vi "GUI_PhasicsHPD.vi"() -> ()   [LabVIEW 2013]
uses:
  shared programs/GUI_Template/GUI_master/tcp_new_data_event.ctl
  shared programs/GUI_Template/GUI_master/tcp new data cluster.ctl
  <vilib>/vision/NI_Vision_Development_Module.lvlib
panel:
  out "Overexposed!":bool
  in  "Tab Control":enum32{"Raw", "Intensity", "Phase"}(tab)
  out "image::1":T1(plugin-control) caption="Raw"
  out "intensityimage::1":T1(plugin-control) caption="Intensity"
  out "phaseimage::1":T1(plugin-control) caption="Phase"
  in  "gain::1":dbl=0.001 caption="gain" min=0.451 max=21.5 format="%_4p"
  in  "exposure::1":dbl=0.001 caption="Exposure" min=0.001 max=1.0 format="%_4p"
  in  "insert tag":bool=TRUE
  in  "stop":bool
  in  "trigger::1":bool caption="Trigger"
  in  "GUIdevice 1":string="U_Phasics"
  out "tcp data event":T2
  out "error IO 2":errorcluster
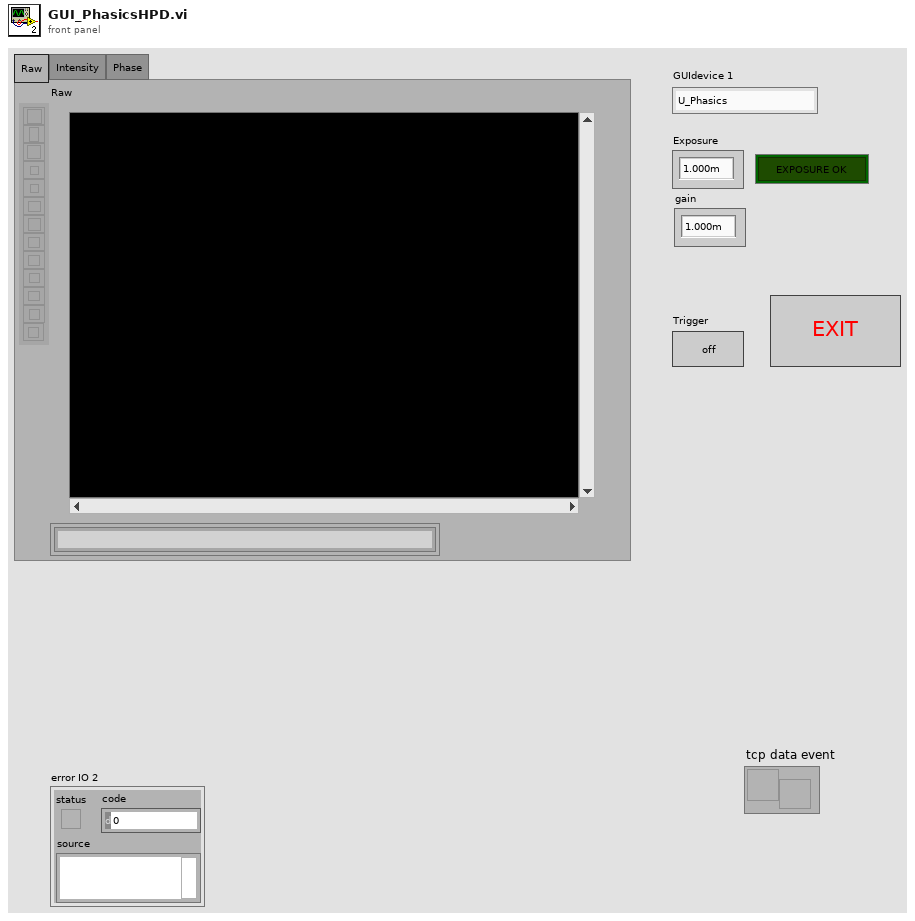
[diagram p1: front panel]
types:
  T1 = typedef "IMAQ Image.ctl" = refnum<image>
  T2 = typedef "tcp_new_data_event.ctl" = refnum<user-event>
  T3 = typedef "Image Type" = u32
  T4 = typedef "tcp new data cluster.ctl" = cluster{"EventEnum":enum16{"new data", "connection status update"}, "Device name":string}
  T5 = cluster{"Starting Value":sgl, "Incremental Value":sgl, "Histogram":u32[]}
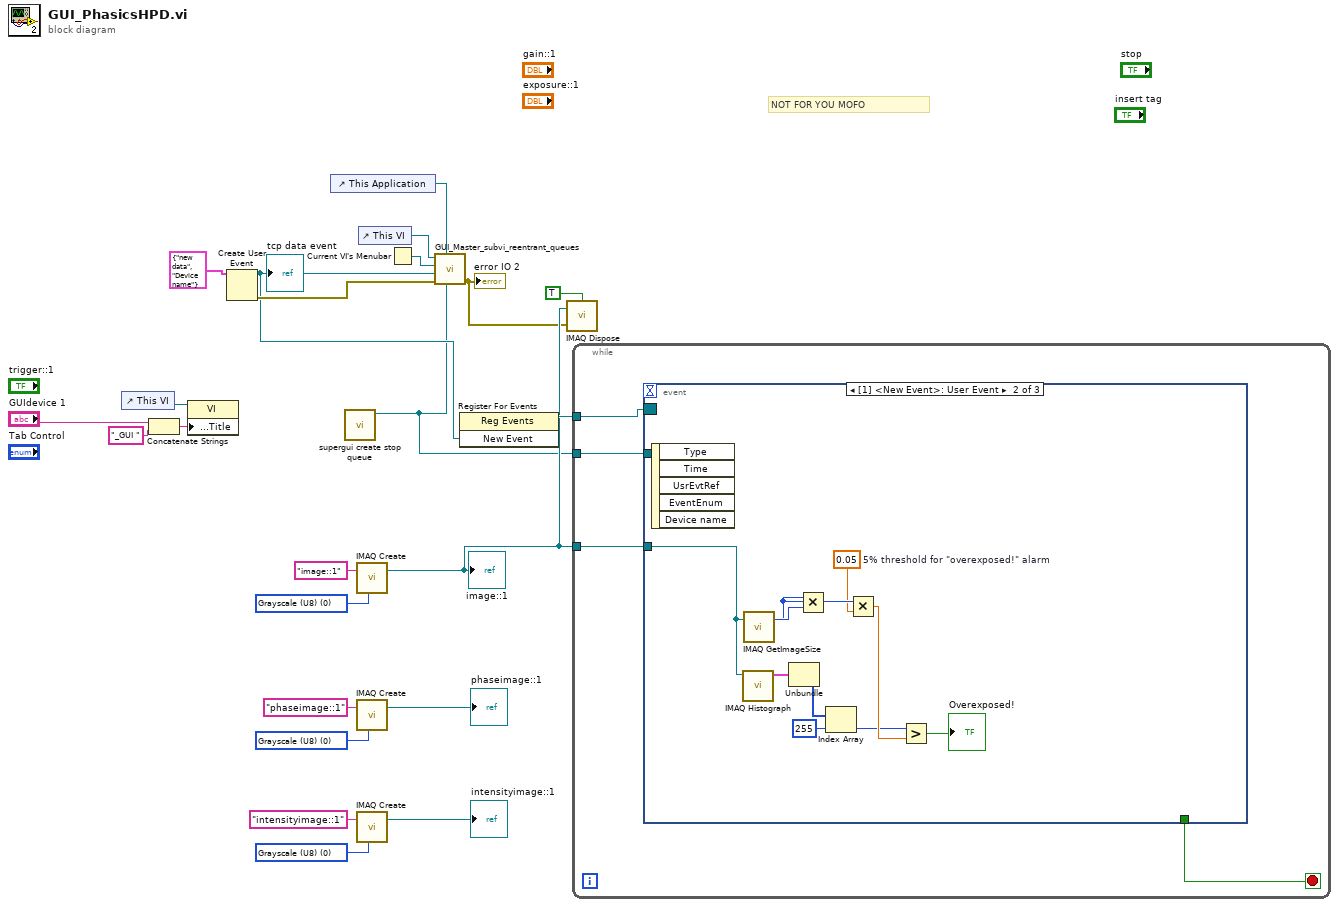
[diagram p0: block diagram]
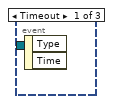
[diagram p2: hidden frame]
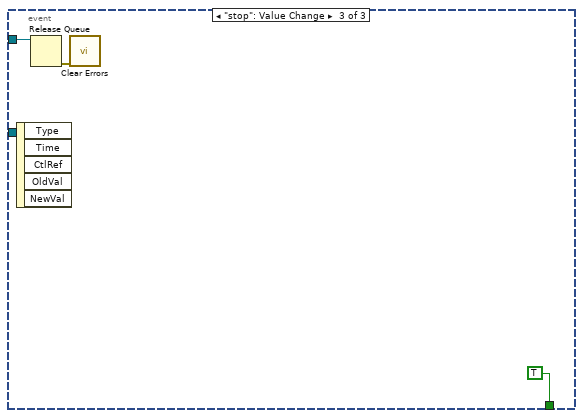
[diagram p3: hidden frame]
diagram:
  w8 = T3 0 items=["Grayscale (U8)", "Grayscale (I16)", "Grayscale (SGL)", "Complex (CSG)", "RGB (U32)", "HSL (U32)", "RGB (U64)", "Grayscale (U16)"] ("Image Type")
  w13 = T3 0 items=["Grayscale (U8)", "Grayscale (I16)", "Grayscale (SGL)", "Complex (CSG)", "RGB (U32)", "HSL (U32)", "RGB (U64)", "Grayscale (U16)"] ("Image Type")
  w16 = T3 0 items=["Grayscale (U8)", "Grayscale (I16)", "Grayscale (SGL)", "Complex (CSG)", "RGB (U32)", "HSL (U32)", "RGB (U64)", "Grayscale (U16)"] ("Image Type")
  # "NOT FOR YOU MOFO"
  n1 = control-ref of="This VI"() -> (w4:refnum<vi>)
  n2 = Concatenate Strings("GUIdevice 1", "_GUI ") -> (w3:string)
  n3 = property class="VI"(reference=w4, "Front Panel.Title"=w3) -> ()  [unwired: 1 in, 2 out]
  n4 = Create User Event(user event datatype=T4 {"EventEnum"=enum."new data", "Device name"="Device name"} ("New Event")) -> (user event=w17:refnum<user-event>, error out=w20:errorcluster)  [unwired: 1 in]
  "tcp data event" <- w17
  n5 = control-ref of="This Application"() -> (w19:refnum<vi>)
  n6 = call "supergui create stop queue.vi"() -> ("STOP Queue out"=w5:refnum<queue>)  [unwired: 11 in]
  n7 = call "IMAQ Create"("Image Name"="image::1", "Image Type"=w13) -> ("New Image"=w12:T1)  [unwired: 3 in, 1 out]
  "image::1" <- w12
  n8 = call "IMAQ Create"("Image Name"="phaseimage::1", "Image Type"=w16) -> ("New Image"=→"phaseimage::1":T1)  [unwired: 3 in, 1 out]
  n9 = call "IMAQ Create"("Image Name"="intensityimage::1", "Image Type"=w8) -> ("New Image"=→"intensityimage::1":T1)  [unwired: 3 in, 1 out]
  n10 = control-ref of="This VI"() -> (w23:refnum<vi>)
  n11 = Current VI's Menubar() -> (w22:refnum<k9>)
  n12 = call "GUI_Master_subvi_reentrant_queues.vi"("STOP Queue in"=w5, "This Application"=w19, "error in (no error)"=w20, "tcp data event"=w17, "Caller menu reference"=w22, "Caller VI ref"=w23) -> ("error out"=w10:errorcluster)  [unwired: 5 in]
  "error IO 2" <- w10
  n13 = register-events(w17) -> (reference out=w18:refnum<event-registration>)  [unwired: 2 in, 1 out]
  n14 = call "IMAQ Dispose"("All Images? (No)"=TRUE, "Image"=w12, "error in (no error)"=w10) -> ()  [unwired: 3 in, 1 out]
  n15 = while {
    tunnel: w18 -> [w26]
    tunnel: w12 -> [w25]
    tunnel: w5 -> [w24]
    stop <- w27 stop-if-true
    n16 = event shown="[1] <New Event>: User Event" {
      selector: w26 -> [_ _ _]
      dyn-events: _ -> [_ _ _]
      timeout: _ -> [_ _ _]
      tunnel: [_ _ TRUE] -> w27
      tunnel: w25 -> [_ w29 _]
      tunnel: w24 -> [_ _ w39]
      event Timeout {
        n17 = event-data() -> ()  [unwired: 1 in, 2 out]
      }
      event User Event {
        w33 = 0.05  # 5% threshold for "overexposed!" alarm
        n18 = event-data() -> ()  [unwired: 1 in, 5 out]
        n19 = call "IMAQ Histograph"("Image"=w29) -> ("Histogram Graph"=w37:T5)  [unwired: 7 in, 3 out]
        n20 = call "IMAQ GetImageSize"("Image"=w29) -> ("Y Resolution"=w35:i32, "X Resolution"=w34:i32)  [unwired: 3 in, 1 out]
        n21 = Unbundle(w37) -> ("Histogram"=w36:u32[])  [unwired: 2 out]
        n22 = Multiply(x=w34, y=w35) -> ()  [unwired: 1 out]
        n23 = Index Array(array=w36, index=255) -> (element=w30:u32)
        n24 = Multiply(x=w34, y=w33) -> (x*y=w31:dbl)
        n25 = Greater?(x=w30, y=w31) -> (0:→"Overexposed!":bool)
      }
      event "stop": Value Change {
        n26 = event-data() -> ()  [unwired: 1 in, 5 out]
        n27 = Release Queue(queue=w39) -> (error out=w38:errorcluster)  [unwired: 2 in, 2 out]
        n28 = call <vilib>:"Clear Errors.vi"("error in (no error)"=w38) -> ()  [unwired: 6 in, 1 out]
      }
    }
  }
